vi "readFile.vi"(8 "error in (no error)":errorcluster, 10 "Path":path=path "/home/ttsai/Documents/stash/ts_tcs_ofc/configData/pinv.esti", 11 "MatOper in":refnum<class "MatOper.lvclass">) -> (0 "error out":errorcluster, 2 "Array":string[](array[string]), 3 "MatOper out":refnum<class "MatOper.lvclass">)   [LabVIEW 2016, in "OfcFunc.lvlib" / "MatOper.lvclass"]
doc: "Read the configuration file by line."
uses:
  MatOper.lvclass
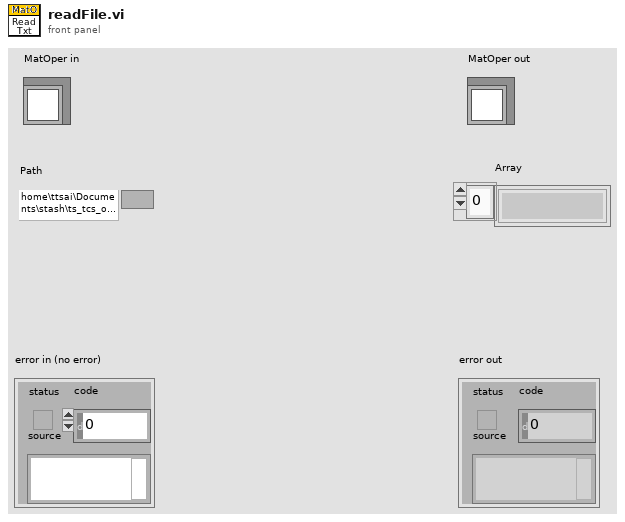
[diagram p1: front panel]
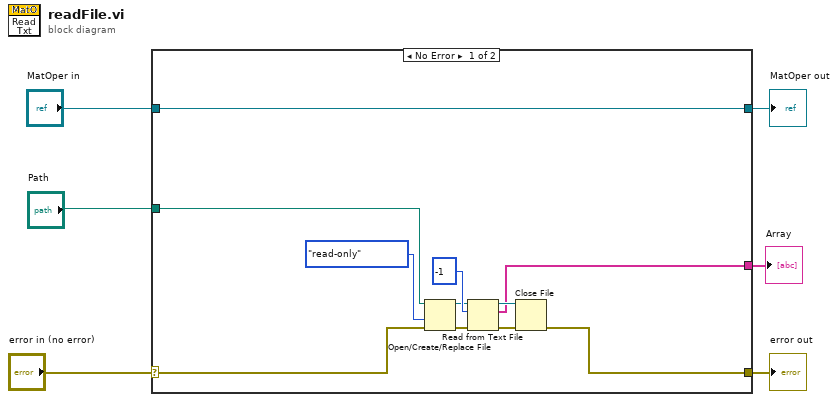
[diagram p0: block diagram]
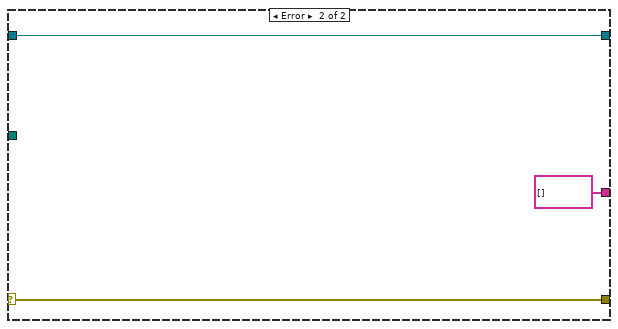
[diagram p2: hidden frame]
diagram:
  n1 = case shown="No Error" "error in (no error)" {
    selector: "error in (no error)" -> [w8 w20]
    tunnel: [w7 w20] -> w5
    tunnel: [w17 w19] -> w3
    tunnel: "MatOper in" -> [w17 w19]
    tunnel: "Path" -> [w10 _]
    tunnel: [w9 string[] []] -> w1
    frame No Error {
      n2 = Open/Create/Replace File(file path (use dialog)=w10, error in=w8, access (0:read/write)=enum16{"read/write", "read-only", "write-only"}."read-only") -> (refnum out=w11:refnum<file>, error out=w13:errorcluster)  [unwired: 3 in, 1 out]
      n3 = Read from Text File(file (use dialog)=w11, count=-1, error in=w13) -> (refnum out=w12:refnum<file>, text=w9:string[], error out=w14:errorcluster)  [unwired: 1 in, 1 out]
      n4 = Close File(refnum=w12, error in=w14) -> (error out=w7:errorcluster)  [unwired: 1 out]
    }
    frame Error {
    }
  }
  "error out" <- w5
  "MatOper out" <- w3
  "Array" <- w1
